vi "GetText.vi"(8 "error in":errorcluster, 11 "Watchdog editor node in":refnum<class "Watchdog editor node.lvclass">) -> (0 "error out":errorcluster, 1 "additional text":string, 2 "text":string, 3 "Watchdog editor node out":refnum<class "Watchdog editor node.lvclass">, 4 "glyph":string)   [LabVIEW 2013, in "Watchdog editor node.lvclass"]
uses:
  Watchdog editor node.lvclass
  <vilib>/NI/DCAF/Tag Editor Core/control module/editor node/control module editor.lvclass
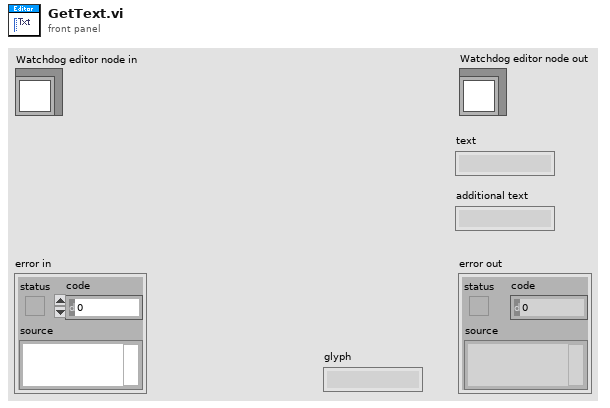
[diagram p1: front panel]
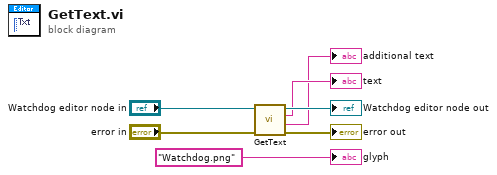
[diagram p0: block diagram]
diagram:
  n1 = call-parent "GetText.vi"("error in"="error in", "Module Editor Node in"="Watchdog editor node in") -> ("error out"=→"error out":errorcluster, "additional text"=→"additional text":string, "text"=→"text":string, "Module Editor Node out"=→"Watchdog editor node out":refnum<class "Watchdog editor node.lvclass">)  [unwired: 5 in, 1 out]
  "glyph" <- "Watchdog.png" ("glyph")
